vi "Mark Result.vi"(8 "error in (no error)":errorcluster, 9 "Complete (F)":bool, 10 "Search Index":i32, 11 "BetterSearch in":refnum<class "BetterSearch.lvclass">) -> (0 "error out":errorcluster, 3 "BetterSearch out":refnum<class "BetterSearch.lvclass">)   [LabVIEW 2016, in "Better Search.lvlib" / "BetterSearch.lvclass"]
uses:
  BetterSearch.lvclass
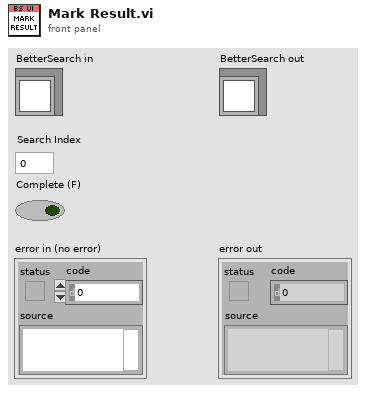
[diagram p1: front panel]
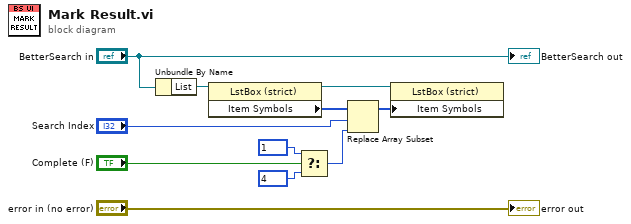
[diagram p0: block diagram]
diagram:
  n1 = Unbundle By Name("BetterSearch in") -> ("List"=w9:refnum<vi>)
  n2 = property class="LstBox (strict)"(reference=w9) -> (reference out=w8:refnum<vi>, "Item Symbols"=w7:i32[])  [unwired: 1 in, 1 out]
  n3 = Select(t=1, s="Complete (F)", f=4) -> (s? t:f=w1:i32)
  n4 = Replace Array Subset(array=w7, new element=w1, index="Search Index") -> (w6:i32[])
  n5 = property class="LstBox (strict)"(reference=w8, "Item Symbols"=w6) -> ()  [unwired: 1 in, 2 out]
  "error out" <- "error in (no error)"
  "BetterSearch out" <- "BetterSearch in"
